vi "SunplusDailyS2TMultiMachineNew.vi"() -> ()   [LabVIEW 2012]
uses:
  <vilib>/addons/database/Auxilliary.llb/DB Tools Cursor Type.ctl
  <vilib>/Utility/NIReport.llb/NI_report.lvclass
  <vilib>/addons/database/Connection.llb/DB Tools Open Connec (Path).vi
  <vilib>/addons/database/Connection.llb/Conn Execute.vi
  <vilib>/addons/database/Recordset.llb/Rec Fetch Recordset Data (R).vi
  <vilib>/addons/database/Recordset.llb/Rec Destroy - Connection.vi
  <vilib>/addons/database/_DB Variant To Data/Database Variant To Data.xnode
  <vilib>/addons/database/NI_Database_API.lvlib
  <vilib>/Utility/NIReport.llb/Excel/NI_Excel.lvclass
  <vilib>/Utility/SMTP/NI_SMTPEmail.lvlib
panel:
  in  "start (0, 0) 4":cluster{"start row":i32, "start column":i32}
  in  "start (0, 0) 3":cluster{"start row":i32, "start column":i32}
  out "error out":errorcluster
  in  "start (0, 0) 2":cluster{"start row":i32, "start column":i32}
  out "error out 2":errorcluster
  in  "MIME content-type (application/octet-stream)":string="application/octet-stream"
  out "error out 4":errorcluster
  in  "start (0, 0)":cluster{"start row":i32, "start column":i32}
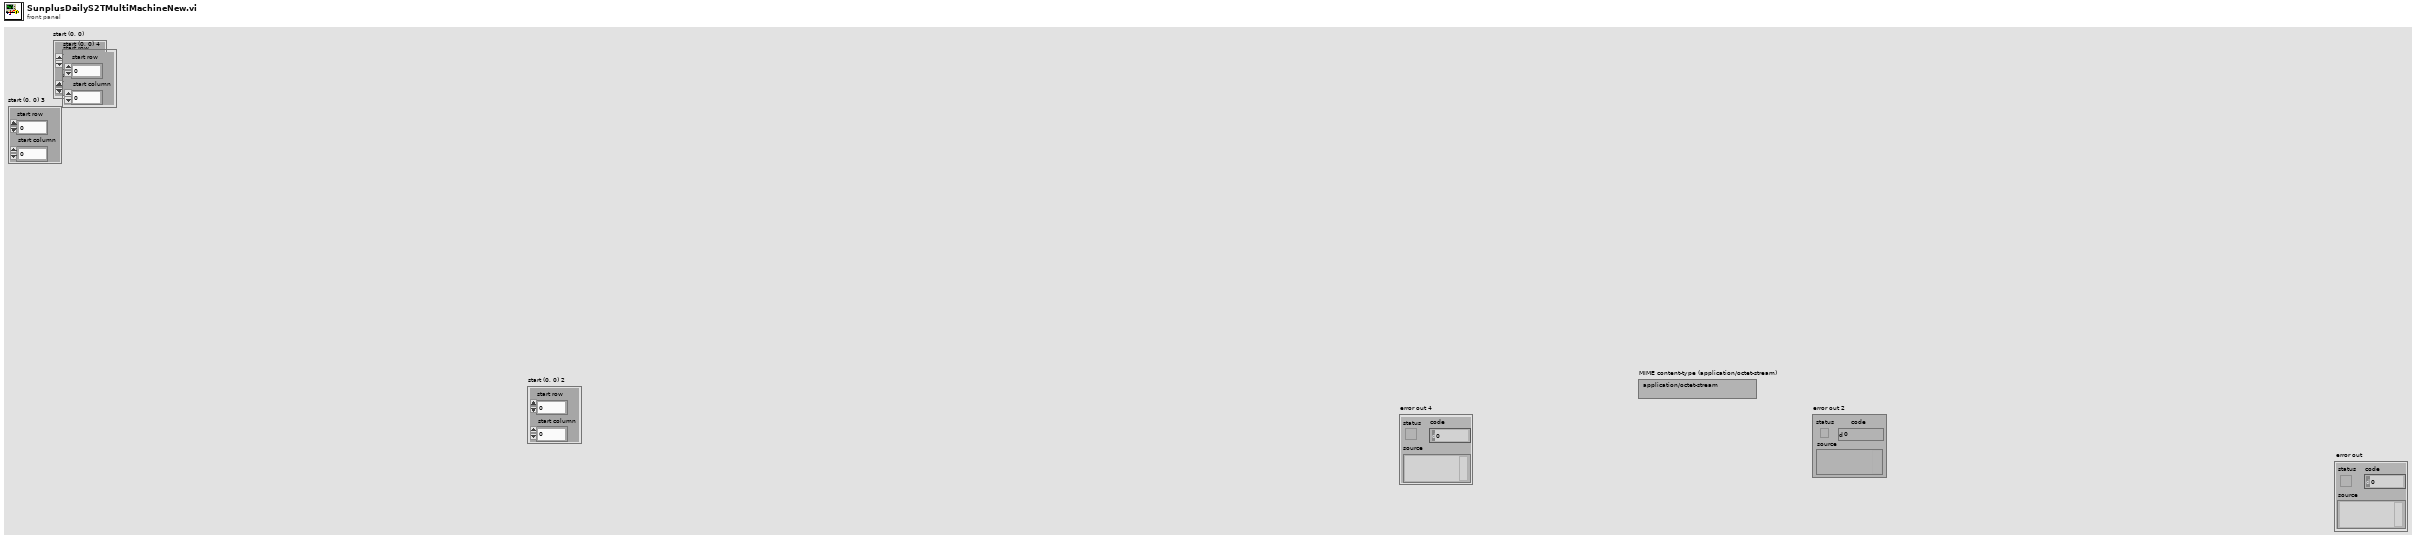
[diagram p1: front panel]
types:
  T1 = typedef "NI_Database_API.lvlib/DB Tools Cursor Type.ctl" = enum16{"forward-only", "keyset", "dynamic", "static"}
  T2 = enum16{"Standard Report", "HTML", "Word", "Excel"}
  T3 = typedef "NI_Database_API.lvlib/Conn ObjectReference.ctl" = refnum<k1>
  T4 = typedef "NI_Database_API.lvlib/Rec ObjectReference.ctl" = refnum<k1>
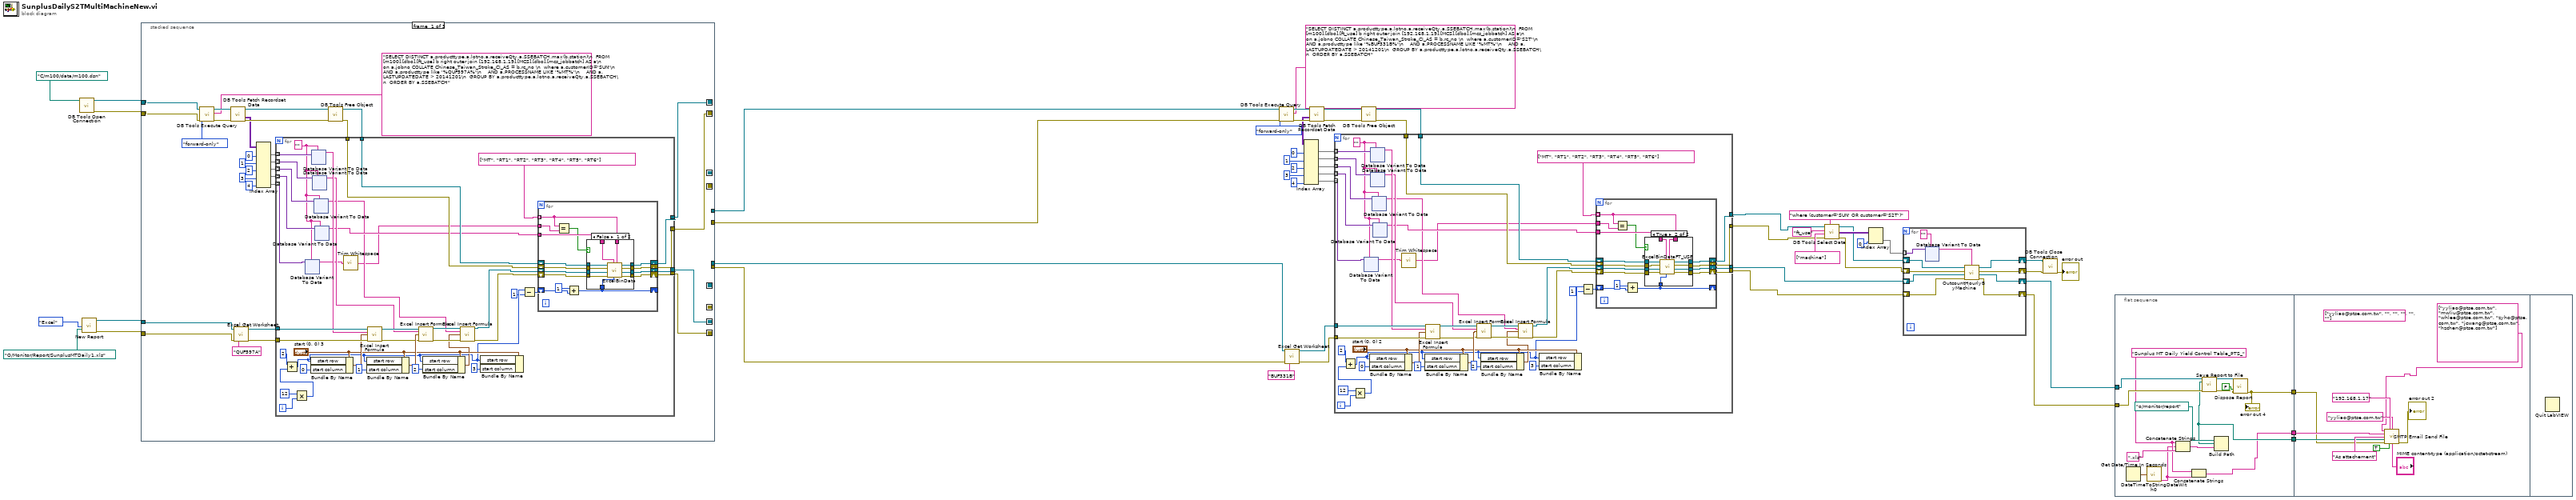
[diagram p0: block diagram]
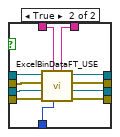
[diagram p2: hidden frame]
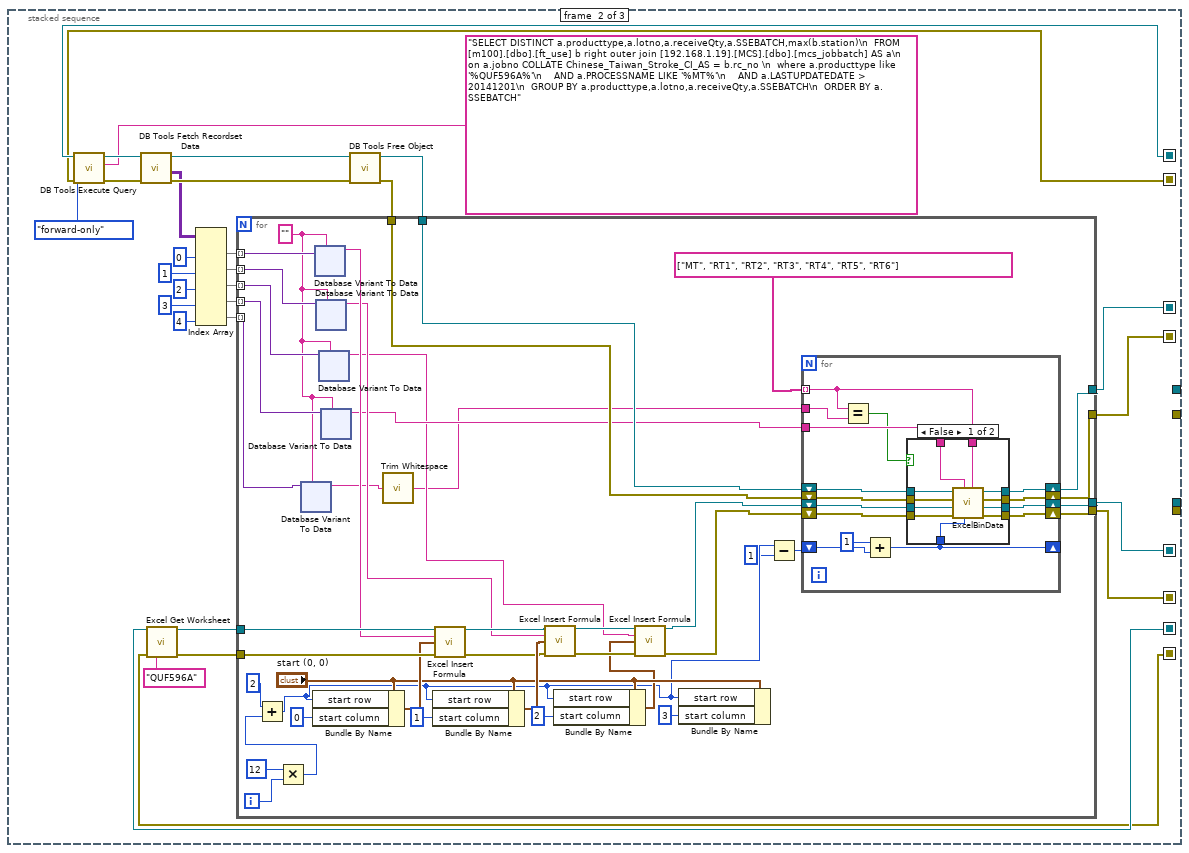
[diagram p3: hidden frame]
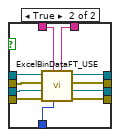
[diagram p4: hidden frame]
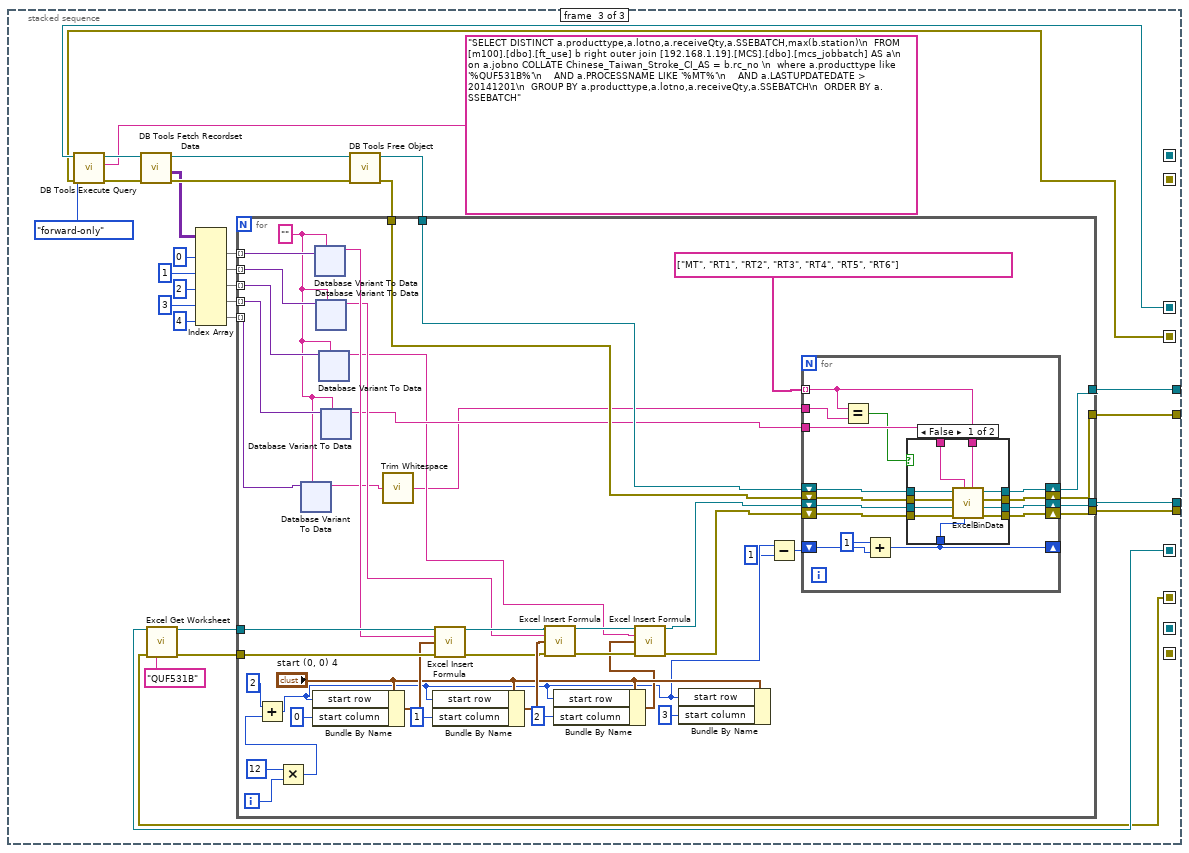
[diagram p5: hidden frame]
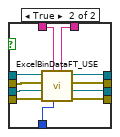
[diagram p6: hidden frame]
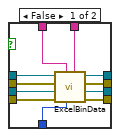
[diagram p7: hidden frame]
diagram:
  n1 = call-poly <vilib>:"DB Tools Open Connection.vi"("connection information"=path "C:/m100/data/m100.dsn") -> ("error out"=w49:errorcluster, "connection reference"=w50:T3)  [unwired: 7 in]
  n2 = call <vilib>:"New Report.vi"("report type"=T2."Excel" ("Report Type"), "template (empty)"=path "O:/Monitor/Report/SunplusMTDaily1.xls") -> ("report out"=w46:refnum<class "NI_report.lvclass">, "error out"=w45:errorcluster)  [unwired: 12 in]
  n3 = stacked-sequence {
    seq-local: [w61 _ _] -> [_ w348 _]
    seq-local: [w60 _ _] -> [_ w347 _]
    seq-local: [w59 _ _] -> [_ w334 _]
    seq-local: [w58 _ _] -> [_ w333 _]
    seq-local: [_ w325 _] -> [_ _ w595]
    seq-local: [_ w326 _] -> [_ _ w594]
    seq-local: [_ w323 _] -> [_ _ w592]
    seq-local: [_ w324 _] -> [_ _ w593]
    tunnel: w50 -> [w57 _ _]
    tunnel: w49 -> [w56 _ _]
    tunnel: w46 -> [w55 _ _]
    tunnel: w45 -> [w54 _ _]
    tunnel: [_ _ w600] -> w38
    tunnel: [_ _ w599] -> w37
    tunnel: [_ _ w598] -> w20
    tunnel: [_ _ w597] -> w19
    frame #0 {
      n4 = call-poly <vilib>:"DB Tools Execute Query.vi"("error in (no error)"=w56, "cursor type"=DB_Tools_Cursor_Type."forward-only", "SQL query"="SELECT DISTINCT a.producttype,a.lotno,a.receiveQty,a.SSEBATCH,max(b.station)\n  FROM [m100].[dbo].[ft_use] b right outer join [192.168.1.19].[MCS].[dbo].[mcs_jobbatch] AS a\n  on a.jobno COLLATE Chinese_Taiwan_Stroke_CI_AS = b.rc_no \n  where a.customerID='SUN'\n    AND a.producttype like '%QUF597A%'\n    AND a.PROCESSNAME LIKE '%MT%'\n    AND a.LASTUPDATEDATE > 20141201\n  GROUP BY a.producttype,a.lotno,a.receiveQty,a.SSEBATCH\n  ORDER BY a.SSEBATCH", "connection reference"=w57) -> ("error out"=w80:errorcluster, "recordset reference"=w81:T4)  [unwired: 4 in]
      n5 = call-poly <vilib>:"DB Tools Fetch Recordset Data.vi"("error in (no error)"=w80, "recordset reference"=w81) -> ("error out"=w82:errorcluster, "recordset data"=w78:variant[][], "recordset reference out"=w83:T4)  [unwired: 3 in]
      n6 = call <vilib>:"Excel Get Worksheet.vi"("report in"=w55, "error in (no error)"=w54, "name (\"\")"="QUF597A" ("name (\"\")")) -> ("report out"=w67:refnum<class "NI_report.lvclass">, "error out"=w66:errorcluster)  [unwired: 11 in]
      n7 = Index Array(array=w78, index (col) #1=0 ("disabled index (col)"), index (col) #2=1 ("index (col)"), index (col) #3=2 ("index (col)"), index (col) #4=3 ("index (col)"), index (col) #5=4 ("index (col)")) -> (element #1=w74:variant[], element #2=w73:variant[], element #3=w72:variant[], element #4=w68:variant[], element #5=w63:variant[])  [unwired: 5 in]
      n8 = call-poly <vilib>:"DB Tools Free Object.vi"("error in (no error)"=w82, "recordset reference"=w83) -> ("error out"=w71:errorcluster, "connection reference"=w70:T3)  [unwired: 8 in]
      n9 = for {
        tunnel: w74 -> [w125] mode=indexing
        tunnel: w73 -> [w124] mode=indexing
        tunnel: w72 -> [w123] mode=indexing
        tunnel: w71 -> [w100]
        tunnel: w70 -> [w101]
        tunnel: w68 -> [w122] mode=indexing
        tunnel: w67 -> [w121]
        tunnel: w66 -> [w120]
        tunnel: [w91] -> w59
        tunnel: [w90] -> w58
        tunnel: [w93] -> w61
        tunnel: [w92] -> w60
        tunnel: w63 -> [w87] mode=indexing
        i -> [w104]
        w86 = ""
        n10 = Multiply(x=12, y=w104) -> (x*y=w102:i32)
        n11 = Add(x=2, y=w102) -> (x+y=w97:i32)
        n12 = xnode "Database Variant To Data"("database variant"=w87, "type"=w86) -> ("data"=w85:string)  [unwired: 1 in, 1 out]
        n13 = Bundle By Name(cluster="start (0, 0) 3", "start row"=w97, "start column"=0) -> (w119:cluster{"start row":i32, "start column":i32})
        n14 = xnode "Database Variant To Data"("database variant"=w125, "type"=w86) -> ("data"=w116:string)  [unwired: 1 in, 1 out]
        n15 = xnode "Database Variant To Data"("database variant"=w124, "type"=w86) -> ("data"=w111:string)  [unwired: 1 in, 1 out]
        n16 = xnode "Database Variant To Data"("database variant"=w123, "type"=w86) -> ("data"=w88:string)  [unwired: 1 in, 1 out]
        n17 = xnode "Database Variant To Data"("database variant"=w122, "type"=w86) -> ("data"=w94:string)  [unwired: 1 in, 1 out]
        n18 = call <vilib>:"Trim Whitespace.vi"("string"=w85) -> ("trimmed string"=w84:string)  [unwired: 1 in]
        n19 = Bundle By Name(cluster="start (0, 0) 3", "start row"=w97, "start column"=1) -> (w114:cluster{"start row":i32, "start column":i32})
        n20 = call <vilib>:"Excel Insert Formula.vi"("report in"=w121, "formula"=w116, "start (0, 0)"=w119, "error in (no error)"=w120) -> ("report out"=w113:refnum<class "NI_report.lvclass">, "error out"=w112:errorcluster)  [unwired: 10 in]
        n21 = call <vilib>:"Excel Insert Formula.vi"("report in"=w113, "formula"=w111, "start (0, 0)"=w114, "error in (no error)"=w112) -> ("report out"=w109:refnum<class "NI_report.lvclass">, "error out"=w108:errorcluster)  [unwired: 10 in]
        n22 = Bundle By Name(cluster="start (0, 0) 3", "start row"=w97, "start column"=2) -> (w105:cluster{"start row":i32, "start column":i32})
        n23 = call <vilib>:"Excel Insert Formula.vi"("report in"=w109, "formula"=w88, "start (0, 0)"=w105, "error in (no error)"=w108) -> ("report out"=w99:refnum<class "NI_report.lvclass">, "error out"=w98:errorcluster)  [unwired: 10 in]
        n24 = Bundle By Name(cluster="start (0, 0) 3", "start row"=w97, "start column"=3) -> ()  [unwired: 1 out]
        n25 = Subtract(x=w97, y=1) -> (x-y=w95:i32)
        n26 = for {
          shift-right: [w171] -> w93
          shift-left: w101 -> [w164]
          shift-right: [w170] -> w92
          shift-left: w100 -> [w163]
          shift-right: [w169] -> w91
          shift-left: w99 -> [w162]
          shift-right: [w168] -> w90
          shift-left: w98 -> [w161]
          shift-right: [w167] -> _
          shift-left: w95 -> [w166]
          tunnel: w94 -> [w165]
          tunnel: string[] ["MT", "RT1", "RT2", "RT3", "RT4", "RT5", "RT6"] ("Array") -> [w159] mode=indexing
          tunnel: w84 -> [w160]
          n27 = Equal?(x=w159, y=w160) -> (x = y?=w158:bool)
          n28 = Add(x=1, y=w166) -> (x+y=w167:i32)
          n29 = case shown="False" w158 {
            tunnel: [w183 w189] -> w171
            tunnel: [w182 w188] -> w170
            tunnel: [w181 w187] -> w169
            tunnel: [w180 w186] -> w168
            tunnel: w167 -> [w179 w194]
            tunnel: w165 -> [w178 w185]
            tunnel: w164 -> [w177 w193]
            tunnel: w163 -> [w176 w192]
            tunnel: w162 -> [w175 w191]
            tunnel: w161 -> [w174 w190]
            tunnel: w159 -> [w173 w184]
            frame False {
              n30 = call "ExcelBinData.vi"("step"=w173, "start row"=w179, "jobno"=w178, "error in (no error) 2"=w174, "report in"=w175, "error in (no error)"=w176, "connection reference 2"=w177) -> ("error out 2"=w180:errorcluster, "report out"=w181:refnum<class "NI_report.lvclass">, "error out"=w182:errorcluster, "connection reference"=w183:T3)  [unwired: 1 in]
            }
            frame True {
              n31 = call "ExcelBinDataFT_USE.vi"("step"=w184, "start row"=w194, "jobno"=w185, "error in (no error) 2"=w190, "report in"=w191, "error in (no error)"=w192, "connection reference 2"=w193) -> ("error out 2"=w186:errorcluster, "report out"=w187:refnum<class "NI_report.lvclass">, "error out"=w188:errorcluster, "connection reference"=w189:T3)  [unwired: 1 in]
            }
          }
        }
      }
    }
    frame #1 {
      n32 = call-poly <vilib>:"DB Tools Execute Query.vi"("error in (no error)"=w347, "cursor type"=DB_Tools_Cursor_Type."forward-only", "SQL query"="SELECT DISTINCT a.producttype,a.lotno,a.receiveQty,a.SSEBATCH,max(b.station)\n  FROM [m100].[dbo].[ft_use] b right outer join [192.168.1.19].[MCS].[dbo].[mcs_jobbatch] AS a\n  on a.jobno COLLATE Chinese_Taiwan_Stroke_CI_AS = b.rc_no \n  where a.producttype like '%QUF596A%'\n    AND a.PROCESSNAME LIKE '%MT%'\n    AND a.LASTUPDATEDATE > 20141201\n  GROUP BY a.producttype,a.lotno,a.receiveQty,a.SSEBATCH\n  ORDER BY a.SSEBATCH", "connection reference"=w348) -> ("error out"=w349:errorcluster, "recordset reference"=w350:T4)  [unwired: 4 in]
      n33 = call-poly <vilib>:"DB Tools Fetch Recordset Data.vi"("error in (no error)"=w349, "recordset reference"=w350) -> ("error out"=w351:errorcluster, "recordset data"=w345:variant[][], "recordset reference out"=w352:T4)  [unwired: 3 in]
      n34 = call <vilib>:"Excel Get Worksheet.vi"("report in"=w334, "error in (no error)"=w333, "name (\"\")"="QUF596A" ("name (\"\")")) -> ("report out"=w332:refnum<class "NI_report.lvclass">, "error out"=w331:errorcluster)  [unwired: 11 in]
      n35 = Index Array(array=w345, index (col) #1=0 ("disabled index (col)"), index (col) #2=1 ("index (col)"), index (col) #3=2 ("index (col)"), index (col) #4=3 ("index (col)"), index (col) #5=4 ("index (col)")) -> (element #1=w341:variant[], element #2=w340:variant[], element #3=w339:variant[], element #4=w335:variant[], element #5=w328:variant[])  [unwired: 5 in]
      n36 = call-poly <vilib>:"DB Tools Free Object.vi"("error in (no error)"=w351, "recordset reference"=w352) -> ("error out"=w338:errorcluster, "connection reference"=w337:T3)  [unwired: 8 in]
      n37 = for {
        tunnel: w341 -> [w394] mode=indexing
        tunnel: w340 -> [w393] mode=indexing
        tunnel: w339 -> [w392] mode=indexing
        tunnel: w338 -> [w369]
        tunnel: w337 -> [w370]
        tunnel: w335 -> [w391] mode=indexing
        tunnel: w332 -> [w390]
        tunnel: w331 -> [w389]
        tunnel: [w360] -> w324
        tunnel: [w359] -> w323
        tunnel: [w362] -> w325
        tunnel: [w361] -> w326
        tunnel: w328 -> [w356] mode=indexing
        i -> [w373]
        w355 = ""
        n38 = Multiply(x=12, y=w373) -> (x*y=w371:i32)
        n39 = Add(x=2, y=w371) -> (x+y=w366:i32)
        n40 = xnode "Database Variant To Data"("database variant"=w356, "type"=w355) -> ("data"=w354:string)  [unwired: 1 in, 1 out]
        n41 = Bundle By Name(cluster="start (0, 0)", "start row"=w366, "start column"=0) -> (w388:cluster{"start row":i32, "start column":i32})
        n42 = xnode "Database Variant To Data"("database variant"=w394, "type"=w355) -> ("data"=w385:string)  [unwired: 1 in, 1 out]
        n43 = xnode "Database Variant To Data"("database variant"=w393, "type"=w355) -> ("data"=w380:string)  [unwired: 1 in, 1 out]
        n44 = xnode "Database Variant To Data"("database variant"=w392, "type"=w355) -> ("data"=w357:string)  [unwired: 1 in, 1 out]
        n45 = xnode "Database Variant To Data"("database variant"=w391, "type"=w355) -> ("data"=w363:string)  [unwired: 1 in, 1 out]
        n46 = call <vilib>:"Trim Whitespace.vi"("string"=w354) -> ("trimmed string"=w353:string)  [unwired: 1 in]
        n47 = Bundle By Name(cluster="start (0, 0)", "start row"=w366, "start column"=1) -> (w383:cluster{"start row":i32, "start column":i32})
        n48 = call <vilib>:"Excel Insert Formula.vi"("report in"=w390, "formula"=w385, "start (0, 0)"=w388, "error in (no error)"=w389) -> ("report out"=w382:refnum<class "NI_report.lvclass">, "error out"=w381:errorcluster)  [unwired: 10 in]
        n49 = call <vilib>:"Excel Insert Formula.vi"("report in"=w382, "formula"=w380, "start (0, 0)"=w383, "error in (no error)"=w381) -> ("report out"=w378:refnum<class "NI_report.lvclass">, "error out"=w377:errorcluster)  [unwired: 10 in]
        n50 = Bundle By Name(cluster="start (0, 0)", "start row"=w366, "start column"=2) -> (w374:cluster{"start row":i32, "start column":i32})
        n51 = call <vilib>:"Excel Insert Formula.vi"("report in"=w378, "formula"=w357, "start (0, 0)"=w374, "error in (no error)"=w377) -> ("report out"=w368:refnum<class "NI_report.lvclass">, "error out"=w367:errorcluster)  [unwired: 10 in]
        n52 = Bundle By Name(cluster="start (0, 0)", "start row"=w366, "start column"=3) -> ()  [unwired: 1 out]
        n53 = Subtract(x=w366, y=1) -> (x-y=w364:i32)
        n54 = for {
          shift-right: [w440] -> w362
          shift-left: w370 -> [w433]
          shift-right: [w439] -> w361
          shift-left: w369 -> [w432]
          shift-right: [w438] -> w360
          shift-left: w368 -> [w431]
          shift-right: [w437] -> w359
          shift-left: w367 -> [w430]
          shift-right: [w436] -> _
          shift-left: w364 -> [w435]
          tunnel: w363 -> [w434]
          tunnel: string[] ["MT", "RT1", "RT2", "RT3", "RT4", "RT5", "RT6"] ("Array") -> [w428] mode=indexing
          tunnel: w353 -> [w429]
          n55 = Equal?(x=w428, y=w429) -> (x = y?=w427:bool)
          n56 = Add(x=1, y=w435) -> (x+y=w436:i32)
          n57 = case shown="False" w427 {
            tunnel: [w452 w458] -> w440
            tunnel: [w451 w457] -> w439
            tunnel: [w450 w456] -> w438
            tunnel: [w449 w455] -> w437
            tunnel: w436 -> [w448 w463]
            tunnel: w434 -> [w447 w454]
            tunnel: w433 -> [w446 w462]
            tunnel: w432 -> [w445 w461]
            tunnel: w431 -> [w444 w460]
            tunnel: w430 -> [w443 w459]
            tunnel: w428 -> [w442 w453]
            frame False {
              n58 = call "ExcelBinData.vi"("step"=w442, "start row"=w448, "jobno"=w447, "error in (no error) 2"=w443, "report in"=w444, "error in (no error)"=w445, "connection reference 2"=w446) -> ("error out 2"=w449:errorcluster, "report out"=w450:refnum<class "NI_report.lvclass">, "error out"=w451:errorcluster, "connection reference"=w452:T3)  [unwired: 1 in]
            }
            frame True {
              n59 = call "ExcelBinDataFT_USE.vi"("step"=w453, "start row"=w463, "jobno"=w454, "error in (no error) 2"=w459, "report in"=w460, "error in (no error)"=w461, "connection reference 2"=w462) -> ("error out 2"=w455:errorcluster, "report out"=w456:refnum<class "NI_report.lvclass">, "error out"=w457:errorcluster, "connection reference"=w458:T3)  [unwired: 1 in]
            }
          }
        }
      }
    }
    frame #2 {
      n60 = call-poly <vilib>:"DB Tools Execute Query.vi"("error in (no error)"=w594, "cursor type"=DB_Tools_Cursor_Type."forward-only", "SQL query"="SELECT DISTINCT a.producttype,a.lotno,a.receiveQty,a.SSEBATCH,max(b.station)\n  FROM [m100].[dbo].[ft_use] b right outer join [192.168.1.19].[MCS].[dbo].[mcs_jobbatch] AS a\n  on a.jobno COLLATE Chinese_Taiwan_Stroke_CI_AS = b.rc_no \n  where a.producttype like '%QUF531B%'\n    AND a.PROCESSNAME LIKE '%MT%'\n    AND a.LASTUPDATEDATE > 20141201\n  GROUP BY a.producttype,a.lotno,a.receiveQty,a.SSEBATCH\n  ORDER BY a.SSEBATCH", "connection reference"=w595) -> ("error out"=w618:errorcluster, "recordset reference"=w619:T4)  [unwired: 4 in]
      n61 = call-poly <vilib>:"DB Tools Fetch Recordset Data.vi"("error in (no error)"=w618, "recordset reference"=w619) -> ("error out"=w620:errorcluster, "recordset data"=w616:variant[][], "recordset reference out"=w621:T4)  [unwired: 3 in]
      n62 = call <vilib>:"Excel Get Worksheet.vi"("report in"=w593, "error in (no error)"=w592, "name (\"\")"="QUF531B" ("name (\"\")")) -> ("report out"=w605:refnum<class "NI_report.lvclass">, "error out"=w604:errorcluster)  [unwired: 11 in]
      n63 = Index Array(array=w616, index (col) #1=0 ("disabled index (col)"), index (col) #2=1 ("index (col)"), index (col) #3=2 ("index (col)"), index (col) #4=3 ("index (col)"), index (col) #5=4 ("index (col)")) -> (element #1=w612:variant[], element #2=w611:variant[], element #3=w610:variant[], element #4=w606:variant[], element #5=w601:variant[])  [unwired: 5 in]
      n64 = call-poly <vilib>:"DB Tools Free Object.vi"("error in (no error)"=w620, "recordset reference"=w621) -> ("error out"=w609:errorcluster, "connection reference"=w608:T3)  [unwired: 8 in]
      n65 = for {
        tunnel: w612 -> [w663] mode=indexing
        tunnel: w611 -> [w662] mode=indexing
        tunnel: w610 -> [w661] mode=indexing
        tunnel: w609 -> [w638]
        tunnel: w608 -> [w639]
        tunnel: w606 -> [w660] mode=indexing
        tunnel: w605 -> [w659]
        tunnel: w604 -> [w658]
        tunnel: [w629] -> w598
        tunnel: [w628] -> w597
        tunnel: [w631] -> w600
        tunnel: [w630] -> w599
        tunnel: w601 -> [w625] mode=indexing
        i -> [w642]
        w624 = ""
        n66 = Multiply(x=12, y=w642) -> (x*y=w640:i32)
        n67 = Add(x=2, y=w640) -> (x+y=w635:i32)
        n68 = xnode "Database Variant To Data"("database variant"=w625, "type"=w624) -> ("data"=w623:string)  [unwired: 1 in, 1 out]
        n69 = Bundle By Name(cluster="start (0, 0) 4", "start row"=w635, "start column"=0) -> (w657:cluster{"start row":i32, "start column":i32})
        n70 = xnode "Database Variant To Data"("database variant"=w663, "type"=w624) -> ("data"=w654:string)  [unwired: 1 in, 1 out]
        n71 = xnode "Database Variant To Data"("database variant"=w662, "type"=w624) -> ("data"=w649:string)  [unwired: 1 in, 1 out]
        n72 = xnode "Database Variant To Data"("database variant"=w661, "type"=w624) -> ("data"=w626:string)  [unwired: 1 in, 1 out]
        n73 = xnode "Database Variant To Data"("database variant"=w660, "type"=w624) -> ("data"=w632:string)  [unwired: 1 in, 1 out]
        n74 = call <vilib>:"Trim Whitespace.vi"("string"=w623) -> ("trimmed string"=w622:string)  [unwired: 1 in]
        n75 = Bundle By Name(cluster="start (0, 0) 4", "start row"=w635, "start column"=1) -> (w652:cluster{"start row":i32, "start column":i32})
        n76 = call <vilib>:"Excel Insert Formula.vi"("report in"=w659, "formula"=w654, "start (0, 0)"=w657, "error in (no error)"=w658) -> ("report out"=w651:refnum<class "NI_report.lvclass">, "error out"=w650:errorcluster)  [unwired: 10 in]
        n77 = call <vilib>:"Excel Insert Formula.vi"("report in"=w651, "formula"=w649, "start (0, 0)"=w652, "error in (no error)"=w650) -> ("report out"=w647:refnum<class "NI_report.lvclass">, "error out"=w646:errorcluster)  [unwired: 10 in]
        n78 = Bundle By Name(cluster="start (0, 0) 4", "start row"=w635, "start column"=2) -> (w643:cluster{"start row":i32, "start column":i32})
        n79 = call <vilib>:"Excel Insert Formula.vi"("report in"=w647, "formula"=w626, "start (0, 0)"=w643, "error in (no error)"=w646) -> ("report out"=w637:refnum<class "NI_report.lvclass">, "error out"=w636:errorcluster)  [unwired: 10 in]
        n80 = Bundle By Name(cluster="start (0, 0) 4", "start row"=w635, "start column"=3) -> ()  [unwired: 1 out]
        n81 = Subtract(x=w635, y=1) -> (x-y=w633:i32)
        n82 = for {
          shift-right: [w709] -> w631
          shift-left: w639 -> [w702]
          shift-right: [w708] -> w630
          shift-left: w638 -> [w701]
          shift-right: [w707] -> w629
          shift-left: w637 -> [w700]
          shift-right: [w706] -> w628
          shift-left: w636 -> [w699]
          shift-right: [w705] -> _
          shift-left: w633 -> [w704]
          tunnel: w632 -> [w703]
          tunnel: string[] ["MT", "RT1", "RT2", "RT3", "RT4", "RT5", "RT6"] ("Array") -> [w697] mode=indexing
          tunnel: w622 -> [w698]
          n83 = Equal?(x=w697, y=w698) -> (x = y?=w696:bool)
          n84 = Add(x=1, y=w704) -> (x+y=w705:i32)
          n85 = case shown="False" w696 {
            tunnel: [w721 w727] -> w709
            tunnel: [w720 w726] -> w708
            tunnel: [w719 w725] -> w707
            tunnel: [w718 w724] -> w706
            tunnel: w705 -> [w717 w732]
            tunnel: w703 -> [w716 w723]
            tunnel: w702 -> [w715 w731]
            tunnel: w701 -> [w714 w730]
            tunnel: w700 -> [w713 w729]
            tunnel: w699 -> [w712 w728]
            tunnel: w697 -> [w711 w722]
            frame False {
              n86 = call "ExcelBinData.vi"("step"=w711, "start row"=w717, "jobno"=w716, "error in (no error) 2"=w712, "report in"=w713, "error in (no error)"=w714, "connection reference 2"=w715) -> ("error out 2"=w718:errorcluster, "report out"=w719:refnum<class "NI_report.lvclass">, "error out"=w720:errorcluster, "connection reference"=w721:T3)  [unwired: 1 in]
            }
            frame True {
              n87 = call "ExcelBinDataFT_USE.vi"("step"=w722, "start row"=w732, "jobno"=w723, "error in (no error) 2"=w728, "report in"=w729, "error in (no error)"=w730, "connection reference 2"=w731) -> ("error out 2"=w724:errorcluster, "report out"=w725:refnum<class "NI_report.lvclass">, "error out"=w726:errorcluster, "connection reference"=w727:T3)  [unwired: 1 in]
            }
          }
        }
      }
    }
  }
  n88 = call-poly <vilib>:"DB Tools Execute Query.vi"("error in (no error)"=w37, "cursor type"=DB_Tools_Cursor_Type."forward-only", "SQL query"="SELECT DISTINCT a.producttype,a.lotno,a.receiveQty,a.SSEBATCH,max(b.station)\n  FROM [m100].[dbo].[ft_use] b right outer join [192.168.1.19].[MCS].[dbo].[mcs_jobbatch] AS a\n  on a.jobno COLLATE Chinese_Taiwan_Stroke_CI_AS = b.rc_no \n  where a.customerID='S2T'\n    AND a.producttype like '%BUF331B%'\n    AND a.PROCESSNAME LIKE '%MT%'\n    AND a.LASTUPDATEDATE > 20141201\n  GROUP BY a.producttype,a.lotno,a.receiveQty,a.SSEBATCH\n  ORDER BY a.SSEBATCH", "connection reference"=w38) -> ("error out"=w40:errorcluster, "recordset reference"=w41:T4)  [unwired: 4 in]
  n89 = call <vilib>:"Excel Get Worksheet.vi"("report in"=w20, "error in (no error)"=w19, "name (\"\")"="BUF331B" ("name (\"\")")) -> ("report out"=w22:refnum<class "NI_report.lvclass">, "error out"=w21:errorcluster)  [unwired: 11 in]
  n90 = call-poly <vilib>:"DB Tools Fetch Recordset Data.vi"("error in (no error)"=w40, "recordset reference"=w41) -> ("error out"=w42:errorcluster, "recordset data"=w31:variant[][], "recordset reference out"=w43:T4)  [unwired: 3 in]
  n91 = Index Array(array=w31, index (col) #1=0 ("disabled index (col)"), index (col) #2=1 ("index (col)"), index (col) #3=2 ("index (col)"), index (col) #4=3 ("index (col)"), index (col) #5=4 ("index (col)")) -> (element #1=w29:variant[], element #2=w28:variant[], element #3=w27:variant[], element #4=w26:variant[], element #5=w25:variant[])  [unwired: 5 in]
  n92 = call-poly <vilib>:"DB Tools Free Object.vi"("error in (no error)"=w42, "recordset reference"=w43) -> ("error out"=w24:errorcluster, "connection reference"=w23:T3)  [unwired: 8 in]
  n93 = for {
    tunnel: w29 -> [w902] mode=indexing
    tunnel: w28 -> [w901] mode=indexing
    tunnel: w27 -> [w900] mode=indexing
    tunnel: w24 -> [w877]
    tunnel: w23 -> [w878]
    tunnel: w26 -> [w899] mode=indexing
    tunnel: w22 -> [w898]
    tunnel: w21 -> [w897]
    tunnel: [w868] -> w8
    tunnel: [w867] -> w7
    tunnel: [w870] -> w9
    tunnel: [w869] -> w10
    tunnel: w25 -> [w864] mode=indexing
    i -> [w881]
    w863 = ""
    n94 = Multiply(x=12, y=w881) -> (x*y=w879:i32)
    n95 = Add(x=2, y=w879) -> (x+y=w874:i32)
    n96 = xnode "Database Variant To Data"("database variant"=w864, "type"=w863) -> ("data"=w862:string)  [unwired: 1 in, 1 out]
    n97 = Bundle By Name(cluster="start (0, 0) 2", "start row"=w874, "start column"=0) -> (w896:cluster{"start row":i32, "start column":i32})
    n98 = xnode "Database Variant To Data"("database variant"=w902, "type"=w863) -> ("data"=w893:string)  [unwired: 1 in, 1 out]
    n99 = xnode "Database Variant To Data"("database variant"=w901, "type"=w863) -> ("data"=w888:string)  [unwired: 1 in, 1 out]
    n100 = xnode "Database Variant To Data"("database variant"=w900, "type"=w863) -> ("data"=w865:string)  [unwired: 1 in, 1 out]
    n101 = xnode "Database Variant To Data"("database variant"=w899, "type"=w863) -> ("data"=w871:string)  [unwired: 1 in, 1 out]
    n102 = call <vilib>:"Trim Whitespace.vi"("string"=w862) -> ("trimmed string"=w861:string)  [unwired: 1 in]
    n103 = Bundle By Name(cluster="start (0, 0) 2", "start row"=w874, "start column"=1) -> (w891:cluster{"start row":i32, "start column":i32})
    n104 = call <vilib>:"Excel Insert Formula.vi"("report in"=w898, "formula"=w893, "start (0, 0)"=w896, "error in (no error)"=w897) -> ("report out"=w890:refnum<class "NI_report.lvclass">, "error out"=w889:errorcluster)  [unwired: 10 in]
    n105 = call <vilib>:"Excel Insert Formula.vi"("report in"=w890, "formula"=w888, "start (0, 0)"=w891, "error in (no error)"=w889) -> ("report out"=w886:refnum<class "NI_report.lvclass">, "error out"=w885:errorcluster)  [unwired: 10 in]
    n106 = Bundle By Name(cluster="start (0, 0) 2", "start row"=w874, "start column"=2) -> (w882:cluster{"start row":i32, "start column":i32})
    n107 = call <vilib>:"Excel Insert Formula.vi"("report in"=w886, "formula"=w865, "start (0, 0)"=w882, "error in (no error)"=w885) -> ("report out"=w876:refnum<class "NI_report.lvclass">, "error out"=w875:errorcluster)  [unwired: 10 in]
    n108 = Bundle By Name(cluster="start (0, 0) 2", "start row"=w874, "start column"=3) -> ()  [unwired: 1 out]
    n109 = Subtract(x=w874, y=1) -> (x-y=w872:i32)
    n110 = for {
      shift-right: [w948] -> w870
      shift-left: w878 -> [w941]
      shift-right: [w947] -> w869
      shift-left: w877 -> [w940]
      shift-right: [w946] -> w868
      shift-left: w876 -> [w939]
      shift-right: [w945] -> w867
      shift-left: w875 -> [w938]
      shift-right: [w944] -> _
      shift-left: w872 -> [w943]
      tunnel: w871 -> [w942]
      tunnel: string[] ["MT", "RT1", "RT2", "RT3", "RT4", "RT5", "RT6"] ("Array") -> [w936] mode=indexing
      tunnel: w861 -> [w937]
      n111 = Equal?(x=w936, y=w937) -> (x = y?=w935:bool)
      n112 = Add(x=1, y=w943) -> (x+y=w944:i32)
      n113 = case shown="True" w935 {
        tunnel: [w960 w966] -> w948
        tunnel: [w959 w965] -> w947
        tunnel: [w958 w964] -> w946
        tunnel: [w957 w963] -> w945
        tunnel: w944 -> [w956 w971]
        tunnel: w942 -> [w955 w962]
        tunnel: w941 -> [w954 w970]
        tunnel: w940 -> [w953 w969]
        tunnel: w939 -> [w952 w968]
        tunnel: w938 -> [w951 w967]
        tunnel: w936 -> [w950 w961]
        frame False {
          n114 = call "ExcelBinData.vi"("step"=w950, "start row"=w956, "jobno"=w955, "error in (no error) 2"=w951, "report in"=w952, "error in (no error)"=w953, "connection reference 2"=w954) -> ("error out 2"=w957:errorcluster, "report out"=w958:refnum<class "NI_report.lvclass">, "error out"=w959:errorcluster, "connection reference"=w960:T3)  [unwired: 1 in]
        }
        frame True {
          n115 = call "ExcelBinDataFT_USE.vi"("step"=w961, "start row"=w971, "jobno"=w962, "error in (no error) 2"=w967, "report in"=w968, "error in (no error)"=w969, "connection reference 2"=w970) -> ("error out 2"=w963:errorcluster, "report out"=w964:refnum<class "NI_report.lvclass">, "error out"=w965:errorcluster, "connection reference"=w966:T3)  [unwired: 1 in]
        }
      }
    }
  }
  n116 = call <vilib>:"DB Tools Select Data.vi"("condition"="where (customer='SUN' OR customer='S2T')", "error in (no error)"=w10, "columns"=string[] ["machine"], "table"="ft_use", "connection reference"=w9) -> ("error out"=w11:errorcluster, "data"=w15:variant[][], "connection reference out"=w12:T3)  [unwired: 1 in]
  n117 = Index Array(array=w15, index (col)=0 ("disabled index (col)")) -> (element=w14:variant[])  [unwired: 1 in]
  n118 = for {
    tunnel: w14 -> [w1109] mode=indexing
    shift-right: [w1103] -> w5
    shift-left: w12 -> [w1101]
    shift-right: [w1102] -> w4
    shift-left: w11 -> [w1100]
    shift-right: [w1106] -> w3
    shift-left: w8 -> [w1110]
    shift-right: [w1105] -> w2
    shift-left: w7 -> [w1104]
    n119 = xnode "Database Variant To Data"("database variant"=w1109, "type"="") -> ("data"=w1107:string)  [unwired: 1 in, 1 out]
    n120 = call "OutcountHourlyByMachine.vi"("Machine"=w1107, "error in (no error) 2"=w1104, "report in"=w1110, "error in (no error)"=w1100, "connection reference"=w1101) -> ("error in (no error) 3"=w1105:errorcluster, "report in 2"=w1106:refnum<class "NI_report.lvclass">, "error out"=w1102:errorcluster, "connection reference 2"=w1103:T3)  [unwired: 3 in]
  }
  n121 = call <vilib>:"DB Tools Close Connection.vi"("error in (no error)"=w4, "connection reference"=w5) -> ("error out"=→"error out":errorcluster)  [unwired: 5 in]
  n122 = flat-sequence {
    tunnel: w3 -> [w1152]
    tunnel: w2 -> [w1151]
    tunnel: [w1143] -> w53
    tunnel: [w1147] -> w52
    tunnel: [w1146] -> w51
    tunnel: w53 -> [w1160]
    tunnel: w52 -> [w1159]
    tunnel: w51 -> [w1158]
    frame #0 {
      w1145 = "Sunplus MT Daily Yield Control Table_PTS_" ("string")
      n123 = Get Date/Time In Seconds() -> (seconds since 1Jan1904=w1149:timestamp)
      n124 = call "DateTimeToStringDateWith0.vi"("time stamp"=w1149) -> ("Dateyyyymmdd"=w1144:string)  [unwired: 9 in, 1 out]
      n125 = Concatenate Strings(w1145, w1144, ".xls" ("string")) -> (w1148:string)
      n126 = Concatenate Strings(w1145, w1144) -> (w1143:string)
      n127 = Build Path(base path=path "o:/monitor/report", name or relative path=w1148) -> (appended path=w1147:path)
      n128 = call-dynamic "Save Report to File.vi"("report in"=w1152, "report file path"=w1147, "error in (no error)"=w1151) -> ("report out"=w1154:refnum<class "NI_report.lvclass">, "error out"=w1153:errorcluster)  [unwired: 11 in]
      n129 = call-dynamic "Dispose Report.vi"("report in"=w1154, "save changes? (F)"=FALSE, "error in (no error)"=w1153) -> ("error out"=w1146:errorcluster)  [unwired: 12 in]
      "error out 4" <- w1146
    }
    frame #1 {
      (unwired) string[] ["yyliao@ptse.com.tw", "", "", "", "", ""] ("recipients")
      n130 = call <vilib>:"SMTP Email Send File.vi"("recipients"=string[] ["yyliao@ptse.com.tw", "mwliu@ptse.com.tw", "whlee@ptse.com.tw", "zyho@ptse.com.tw", "jcwang@ptse.com.tw", "hzchen@ptse.com.tw"], "mail server"="192.168.1.17", "return address"="yyliao@ptse.com.tw", "subject ([No Subject])"=w1160, "message"="As attachement", "file path"=w1159, "error in (no error)"=w1158, "binary? (F)"=TRUE, "MIME content-type (application/octet-stream)"="MIME content-type (application/octet-stream)") -> ("error out"=→"error out 2":errorcluster)  [unwired: 5 in, 1 out]
    }
    frame #2 {
      n131 = Quit LabVIEW() -> ()  [unwired: 1 in]
    }
  }
